vi "Main.vi"() -> ()   [LabVIEW 2020]
uses:
  <vilib>/Utility/error.llb/DialogType.ctl
  <vilib>/DAQmx/read.llb/DAQmx Read (Analog 1D Wfm NChan NSamp).vi
  <extravilib>/ChannelInstances/Tag-bool/Write With Abort.vi
  <extravilib>/ChannelInstances/Tag-bool/Read With Abort.vi
  <extravilib>/ChannelInstances/Tag-bool/Instantiate.vi
  <vilib>/DAQmx/create/channels.llb/DAQmx Create Channel (AI-Acceleration-Accelerometer).vi
  <vilib>/DAQmx/configure/timing.llb/DAQmx Timing (Sample Clock).vi
  <extravilib>/ChannelInstances/Tag-bool/EndpointRead.vi
  <vilib>/DAQmx/miscellaneous.llb/DAQmx Fill In Error Info.vi
  <vilib>/Waveform/DWDTOps.llb/DWDT Digital to Analog.vi
  <vilib>/ULx/Create Channel.llb/ULx Create Channel (AI-Voltage-Basic).vi
  <vilib>/ULx/Timing.llb/ULx Timing (Sample Clock).vi
  <vilib>/ULx/Read.llb/ULx Read (Analog 1D Wfm NChan NSamp).vi
  <vilib>/DAQmx/create/channels.llb/DAQmx Create Channel (CO-Pulse Generation-Frequency).vi
  <vilib>/DAQmx/configure/timing.llb/DAQmx Timing (Implicit).vi
  <extravilib>/ChannelInstances/Tag-bool/Endpoint.vi
  <extravilib>/ChannelInstances/Tag-bool.lvlib
panel:
  in  "Accels":bool
  in  "Tach":bool
  in  "Mic Enable":bool
  in  "Load Enable":bool
  in  "Encoder Enable":bool
  in  "Torque/Power Enable":bool
  in  "Doppler":bool
  out "Feet Traveled":u64
  out "Power":dynamicdata(graph)
  out "Rev Count":u16
  out "Torque":dynamicdata(graph)
  out "Tach Graph":digitalwaveform[](graph)
  out "Accel Graph":waveform(dbl)[](graph)
  out "Microphones":dynamicdata(graph)
  out "Load Cell Graph":waveform(dbl)[](graph)
  in  "stop":bool
  # "Doppler Speed Sensor"
  # "Torque Encoder"
  # "Operation Instructions: Use the toggle buttons to turn on/off the data acquisition for the various sensors. The Power and Torque are aquired together so toggling the Torque button will also toggle Power.\nPress Run from the toolbar (ctrl + r) to start acquisition and press the Stop key to end aquisition. Make sure sensor power supplies are on!!!"
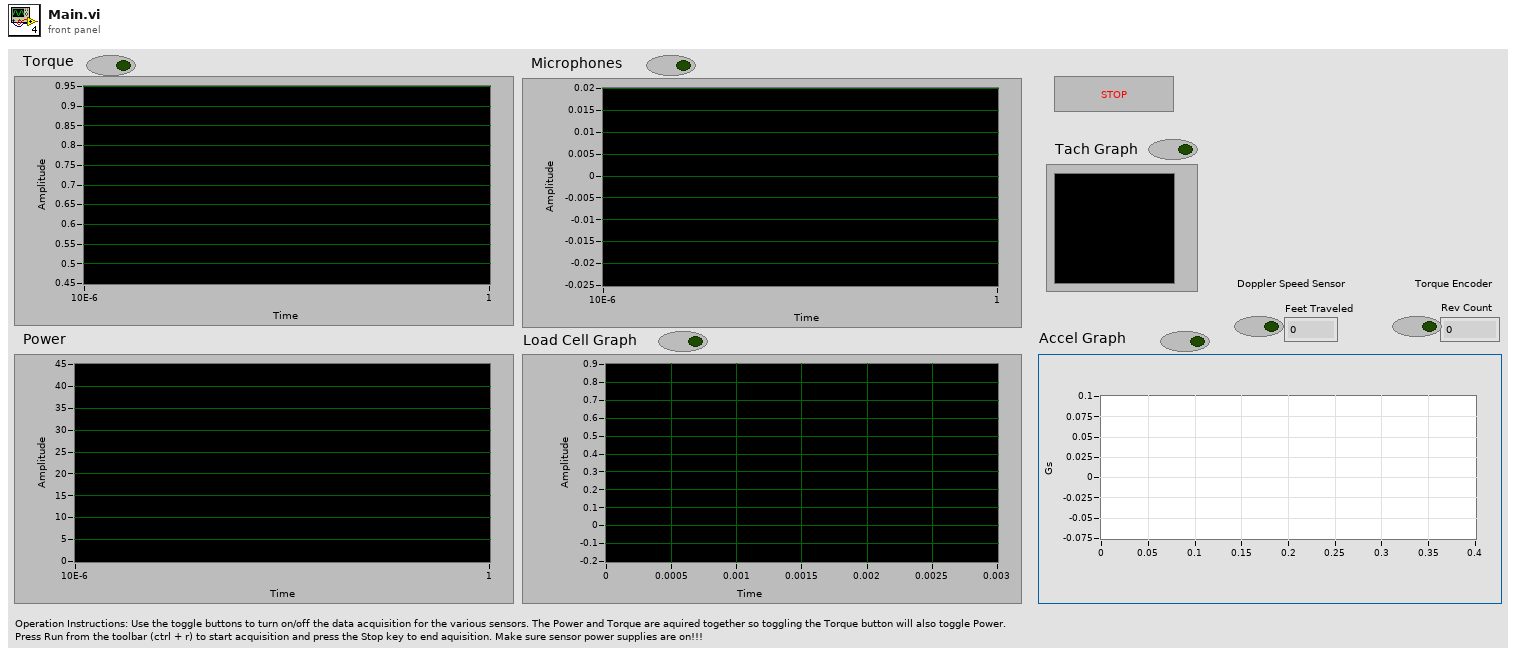
[diagram p1: front panel]
types:
  T1 = typedef "DialogType.ctl" = u16
  T2 = typedef "Tag-bool.lvlib/))Channel.ctl" = refnum<queue>
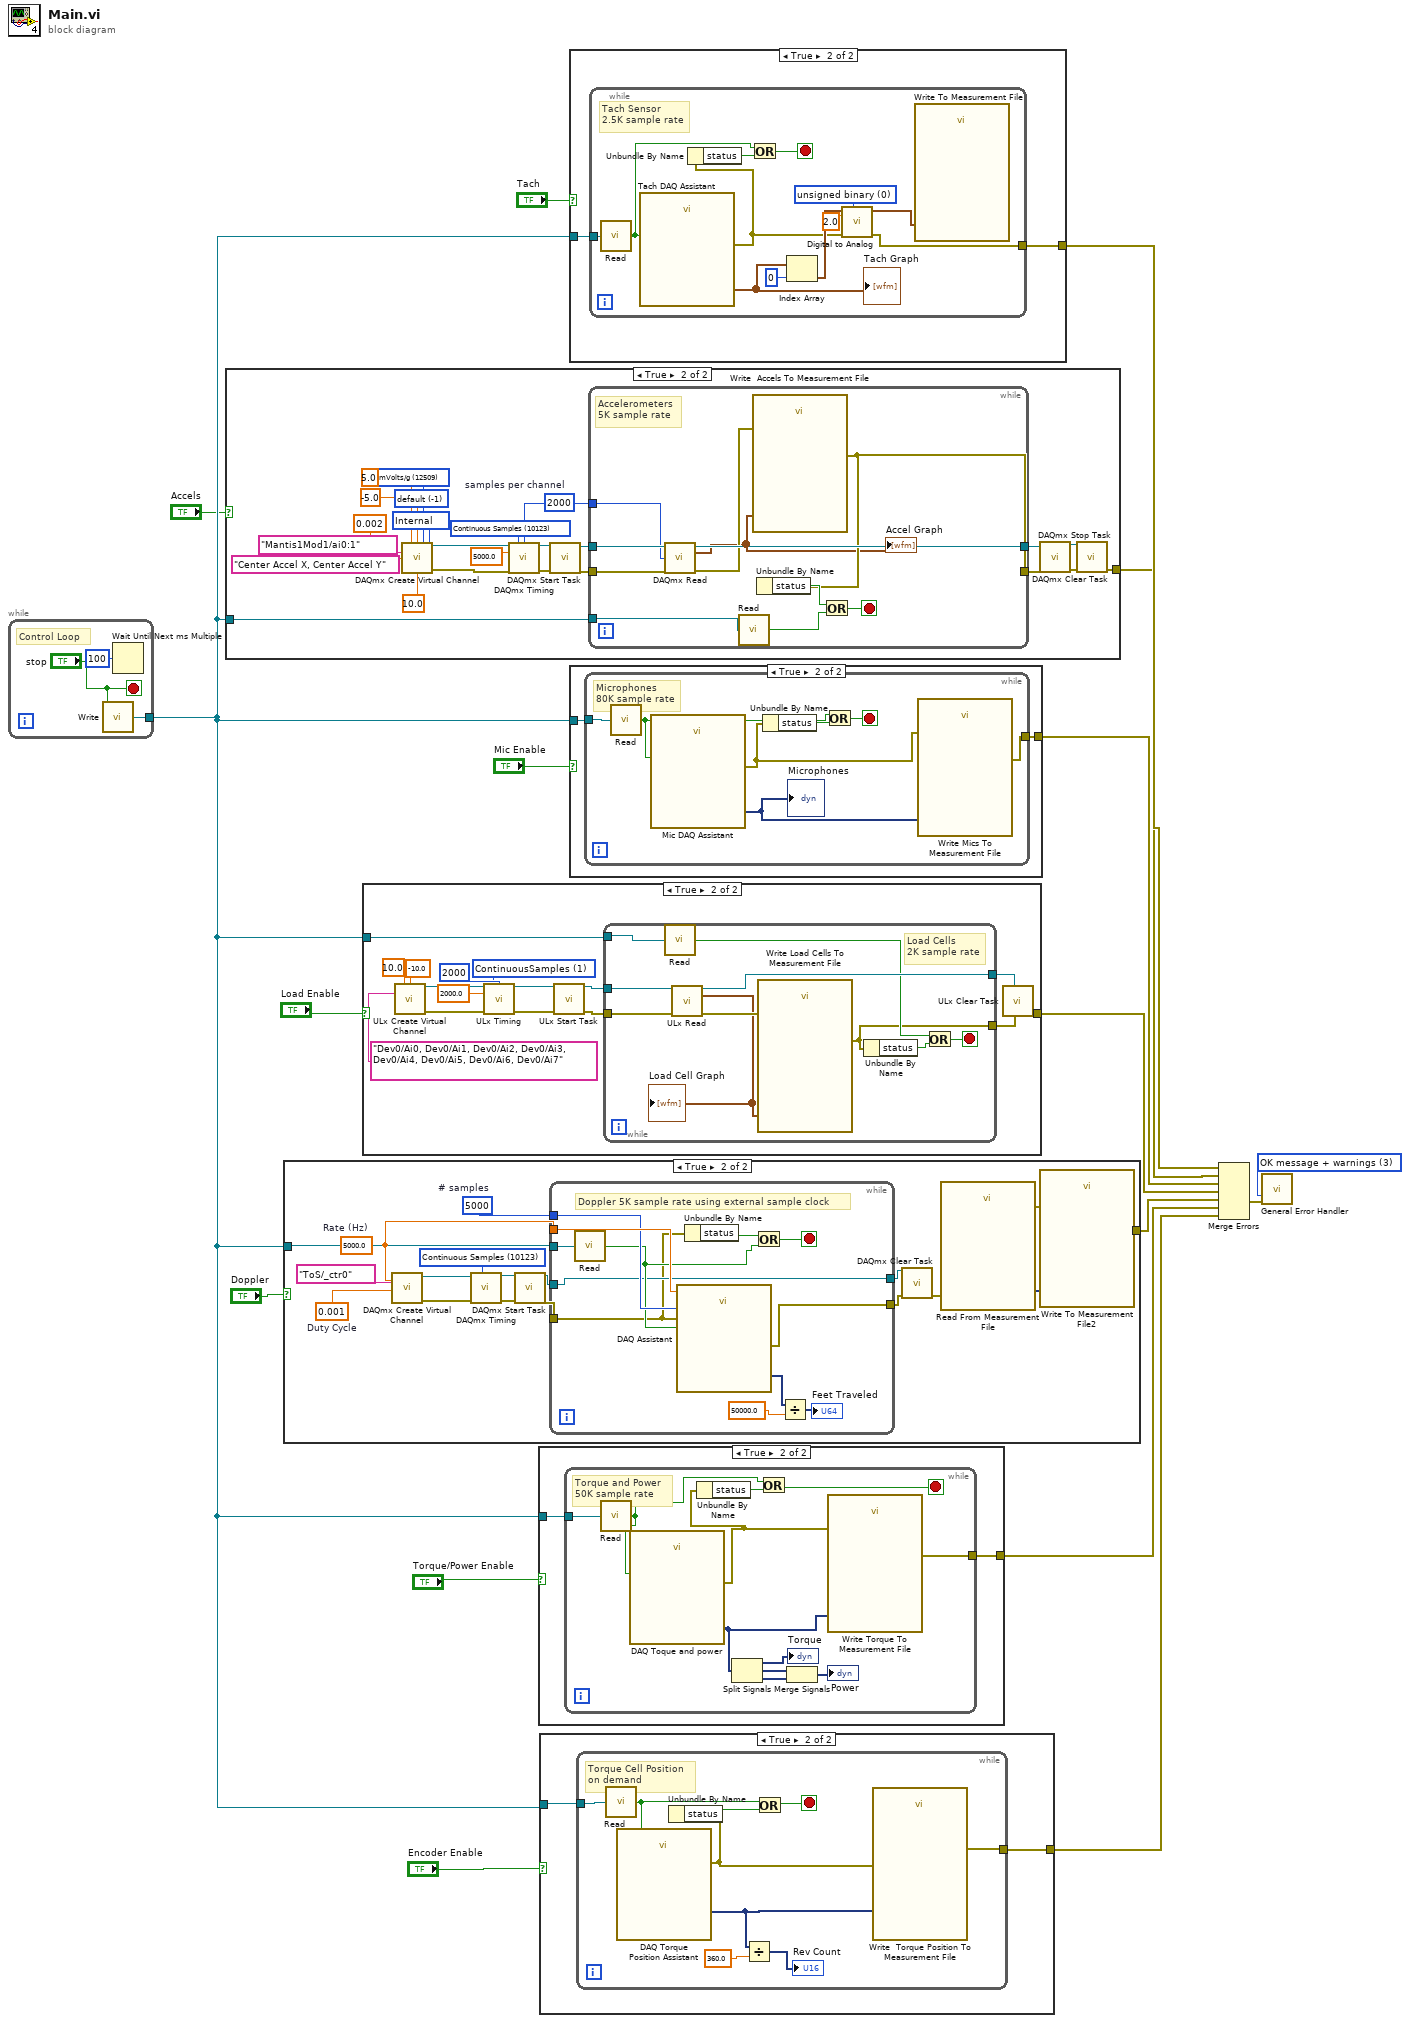
[diagram p0: block diagram]
diagram:
  w17 = T1 3 items=["no dialog", "OK message", "continue or stop message", "OK message + warnings", "continue/stop + warnings"] ("type of dialog (OK msg:1)")
  n1 = while {
    tunnel: [w18] -> w16
    stop <- "stop" stop-if-true
    # "Control Loop"
    n2 = call <extravilib>:"Write.vi"("element"="stop") -> ("channel"=w18:T2)  [unwired: 1 out]
    n3 = Wait Until Next ms Multiple(millisecond multiple=u32 100 ("millisecond timer value")) -> ()  [unwired: 1 out]
  }
  n4 = case shown="True" "Accels" {
    tunnel: w16 -> [_ w22]
    tunnel: [_ w21] -> w7
    frame False {
    }
    frame True {
      w26 = 12509 items=["mVolts/g"=12509, "Volts/g"=12510] ("sensitivity units")
      w29 = 10200 items=["Internal"=10200, "External"=10167, "None"=10230] ("current excitation source")
      w30 = -1 items=["default"=-1, "RSE"=10083, "NRSE"=10078, "Differential"=10106, "Pseudodifferential"=12529] ("input terminal configuration")
      w34 = 2000  # samples per channel
      w42 = 10123 items=["Finite Samples"=10178, "Continuous Samples"=10123, "Hardware Timed Single Point"=12522] ("Sample Mode")
      n5 = call-poly <vilib>:"DAQmx Create Virtual Channel.vi"("maximum value"=5.0, "minimum value"=-5.0, "input terminal configuration"=w30, "physical channels"=tag "Mantis1Mod1/ai0:1", "current excitation source"=w29, "name to assign"="Center Accel X, Center Accel Y", "current excitation value"=0.002, "sensitivity"=10.0, "sensitivity units"=w26) -> ("task out"=w24:refnum<k21>, "error out"=w23:errorcluster)  [unwired: 5 in]
      n6 = call-poly <vilib>:"DAQmx Timing.vi"("task/channels in"=w24, "sample mode"=w42, "samples per channel"=w34, "rate"=5000.0, "error in"=w23) -> ("task out"=w44:refnum<k21>, "error out"=w43:errorcluster)  [unwired: 9 in]
      n7 = call <vilib>:"DAQmx Start Task.vi"("task/channels in"=w44, "error in"=w43) -> ("task out"=w41:refnum<k21>, "error out"=w40:errorcluster)  [unwired: 12 in]
      n8 = while {
        tunnel: w41 -> [w55]
        tunnel: w40 -> [w54]
        tunnel: [w53] -> w39
        tunnel: [w46] -> w38
        tunnel: w34 -> [w50]
        tunnel: w22 -> [w48]
        stop <- w51 stop-if-true
        # "Accelerometers\n5K sample rate"
        n9 = call-poly <vilib>:"DAQmx Read.vi"("task/channels in"=w55, "number of samples per channel"=w50, "error in"=w54) -> ("task out"=w53:refnum<k21>, "data"=w45:waveform(dbl)[], "error out"=w47:errorcluster)  [unwired: 10 in]
        "Accel Graph" <- w45
        n10 = call <extravilib>:"Read.vi"("channel"=w48) -> ("element"=w49:bool)  [unwired: 1 in, 1 out]
        n11 = call "Write  Accels To Measurement File"("Signals"=w45, "error in (no error)"=w47) -> ("error out"=w46:errorcluster)  [unwired: 15 in, 2 out]
        n12 = Unbundle By Name(w46) -> ("status"=w52:bool)
        n13 = Or(x=w52, y=w49) -> (x .or. y?=w51:bool)
      }
      n14 = call <vilib>:"DAQmx Stop Task.vi"("task/channels in"=w39, "error in"=w38) -> ("task out"=w36:refnum<k21>, "error out"=w37:errorcluster)  [unwired: 12 in]
      n15 = call <vilib>:"DAQmx Clear Task.vi"("task in"=w36, "error in"=w37) -> ("error out"=w21:errorcluster)  [unwired: 13 in]
    }
  }
  n16 = case shown="True" "Doppler" {
    tunnel: w16 -> [_ w66]
    tunnel: [_ w59] -> w2
    frame False {
    }
    frame True {
      w68 = 5000  # # samples
      w56 = 5000.0  # Rate (Hz)
      w69 = 0.001  # Duty Cycle
      w71 = 10123 items=["Finite Samples"=10178, "Continuous Samples"=10123] ("sample mode")
      n17 = call-poly <vilib>:"DAQmx Create Virtual Channel.vi"("frequency"=w56, "duty cycle"=w69, "counter"=tag "ToS/_ctr0" ("Sample Clock Src")) -> ("task out"=w72:refnum<k21>, "error out"=w73:errorcluster)  [unwired: 11 in]
      n18 = call-poly <vilib>:"DAQmx Timing.vi"("task/channels in"=w72, "sample mode"=w71, "error in"=w73) -> ("task out"=w58:refnum<k21>, "error out"=w57:errorcluster)  [unwired: 11 in]
      n19 = call <vilib>:"DAQmx Start Task.vi"("task/channels in"=w58, "error in"=w57) -> ("task out"=w63:refnum<k21>, "error out"=w61:errorcluster)  [unwired: 12 in]
      n20 = while {
        tunnel: w56 -> [w85]
        tunnel: w68 -> [w83]
        tunnel: [w81] -> w67
        tunnel: w66 -> [w76]
        tunnel: w63 -> [w75]
        tunnel: [w75] -> w62
        tunnel: w61 -> [w74]
        stop <- w82 stop-if-true
        # "Doppler 5K sample rate using external sample clock"
        n21 = call <extravilib>:"Read.vi"("channel"=w76) -> ("element"=w77:bool)  [unwired: 1 in, 1 out]
        n22 = call "DAQ Assistant"("rate"=w85, "number of samples"=w83, "error in"=w74, "stop (F)"=w77) -> ("data"=w79:dynamicdata, "error out"=w81:errorcluster)  [unwired: 12 in, 2 out]
        n23 = Unbundle By Name(w74) -> ("status"=w84:bool)
        n24 = Or(x=w84, y=w77) -> (x .or. y?=w82:bool)
        n25 = Divide(x=w79, y=50000.0) -> (x/y=→"Feet Traveled":dynamicdata)
      }
      n26 = call <vilib>:"DAQmx Clear Task.vi"("task in"=w62, "error in"=w67) -> ("error out"=w60:errorcluster)  [unwired: 13 in]
      n27 = call "Read From Measurement File"("error in (no error)"=w60) -> ("error out"=w64:errorcluster, "Signals"=w65:dynamicdata)  [unwired: 5 in, 4 out]
      n28 = call "Write To Measurement File2"("Signals"=w65, "error in (no error)"=w64) -> ("error out"=w59:errorcluster)  [unwired: 15 in, 2 out]
    }
  }
  n29 = case shown="True" "Load Enable" {
    tunnel: w16 -> [_ w87]
    tunnel: [_ w86] -> w14
    frame False {
    }
    frame True {
      w94 = 1 items=["FiniteSamples", "ContinuousSamples"] ("sample mode")
      n30 = call-poly <vilib>:"ULx Create Virtual Channel.vi"("maximum value"=10.0, "minimum value"=-10.0, "physical channels"="Dev0/Ai0, Dev0/Ai1, Dev0/Ai2, Dev0/Ai3, Dev0/Ai4, Dev0/Ai5, Dev0/Ai6, Dev0/Ai7") -> ("task out"=w99:refnum<k24>, "error out"=w101:errorcluster)  [unwired: 11 in]
      n31 = call-poly <vilib>:"ULx Timing.vi"("task in"=w99, "sample mode"=w94, "samples per channel"=2000, "rate"=2000.0, "error in"=w101) -> ("task out"=w90:refnum<k24>, "error out"=w97:errorcluster)  [unwired: 9 in]
      n32 = call <vilib>:"ULx Start Task.vi"("task in"=w90, "error in"=w97) -> ("task out"=w98:refnum<k24>, "error out"=w100:errorcluster)  [unwired: 12 in]
      n33 = while {
        tunnel: w100 -> [w108]
        tunnel: w98 -> [w111]
        tunnel: [w110] -> w89
        tunnel: w87 -> [w107]
        tunnel: [w103] -> w88
        stop <- w109 stop-if-true
        # "Load Cells\n2K sample rate"
        n34 = call <extravilib>:"Read.vi"("channel"=w107) -> ("element"=w105:bool)  [unwired: 1 in, 1 out]
        n35 = call-poly <vilib>:"ULx Read.vi"("task in"=w111, "error in"=w108) -> ("task out"=w110:refnum<k24>, "data"=w102:waveform(dbl)[], "error out"=w104:errorcluster)  [unwired: 11 in]
        "Load Cell Graph" <- w102
        n36 = call "Write Load Cells To Measurement File"("Signals"=w102, "error in (no error)"=w104) -> ("error out"=w103:errorcluster)  [unwired: 15 in, 2 out]
        n37 = Unbundle By Name(w103) -> ("status"=w106:bool)
        n38 = Or(x=w105, y=w106) -> (x .or. y?=w109:bool)
      }
      n39 = call <vilib>:"ULx Clear Task.vi"("task in"=w89, "error in"=w88) -> ("error out"=w86:errorcluster)  [unwired: 13 in]
    }
  }
  n40 = case shown="True" "Torque/Power Enable" {
    tunnel: w16 -> [_ w113]
    tunnel: [_ w112] -> w1
    frame False {
    }
    frame True {
      n41 = while {
        tunnel: w113 -> [w124]
        tunnel: [w119] -> w112
        stop <- w122 stop-if-true
        # "Torque and Power\n50K sample rate"
        n42 = call <extravilib>:"Read.vi"("channel"=w124) -> ("element"=w121:bool)  [unwired: 1 in, 1 out]
        n43 = call "DAQ Toque and power"("stop (F)"=w121) -> ("data"=w118:dynamicdata, "error out"=w120:errorcluster)  [unwired: 15 in, 2 out]
        n44 = Unbundle By Name(w120) -> ("status"=w123:bool)
        n45 = Split Signals(w118) -> (→"Torque":dynamicdata, w116:dynamicdata, w115:dynamicdata)  [unwired: 3 in]
        n46 = Or(x=w121, y=w123) -> (x .or. y?=w122:bool)
        n47 = Merge Signals(w116, w115) -> (→"Power":dynamicdata)
        n48 = call "Write Torque To Measurement File"("Signals"=w118, "error in (no error)"=w120) -> ("error out"=w119:errorcluster)  [unwired: 15 in, 2 out]
      }
    }
  }
  n49 = case shown="True" "Encoder Enable" {
    tunnel: w16 -> [_ w126]
    tunnel: [_ w125] -> w13
    frame False {
    }
    frame True {
      n50 = while {
        tunnel: w126 -> [w131]
        tunnel: [w130] -> w125
        stop <- w135 stop-if-true
        # "Torque Cell Position\non demand"
        n51 = call <extravilib>:"Read.vi"("channel"=w131) -> ("element"=w132:bool)  [unwired: 1 in, 1 out]
        n52 = call "DAQ Torque Position Assistant"("stop (F)"=w132) -> ("data"=w129:dynamicdata, "error out"=w133:errorcluster)  [unwired: 15 in, 2 out]
        n53 = Unbundle By Name(w133) -> ("status"=w134:bool)
        n54 = Divide(x=w129, y=360.0) -> (x/y=→"Rev Count":dynamicdata)
        n55 = Or(x=w132, y=w134) -> (x .or. y?=w135:bool)
        n56 = call "Write  Torque Position To Measurement File"("Signals"=w129, "error in (no error)"=w133) -> ("error out"=w130:errorcluster)  [unwired: 15 in, 2 out]
      }
    }
  }
  n57 = case shown="True" "Tach" {
    tunnel: w16 -> [_ w137]
    tunnel: [_ w136] -> w8
    frame False {
    }
    frame True {
      n58 = while {
        tunnel: w137 -> [w149]
        tunnel: [w140] -> w136
        stop <- w148 stop-if-true
        w142 = u16 0 items=["unsigned binary", "offset binary", "2's complement"] ("data format (offset binary)")
        # "Tach Sensor\n2.5K sample rate"
        n59 = call <extravilib>:"Read.vi"("channel"=w149) -> ("element"=w146:bool)  [unwired: 1 in, 1 out]
        n60 = call "Tach DAQ Assistant"("stop (F)"=w146) -> ("data"=w145:digitalwaveform[], "error out"=w141:errorcluster)  [unwired: 15 in, 2 out]
        "Tach Graph" <- w145
        n61 = Unbundle By Name(w141) -> ("status"=w147:bool)
        n62 = Or(x=w146, y=w147) -> (x .or. y?=w148:bool)
        n63 = Index Array(array=w145, index=0) -> (element=w143:digitalwaveform)
        n64 = call-poly <vilib>:"Digital to Analog.vi"("data format (offset binary)"=w142, "error in (no error)"=w141, "full-scale range (pk-pk)"=2.0, "digital waveform"=w143) -> ("error out"=w140:errorcluster, "analog waveform"=w139:waveform(dbl))  [unwired: 4 in, 2 out]
        n65 = call "Write To Measurement File"("Signals"=w139) -> ()  [unwired: 16 in, 3 out]
      }
    }
  }
  n66 = case shown="True" "Mic Enable" {
    tunnel: w16 -> [_ w151]
    tunnel: [_ w150] -> w6
    frame False {
    }
    frame True {
      n67 = while {
        tunnel: w151 -> [w158]
        tunnel: [w154] -> w150
        stop <- w157 stop-if-true
        # "Microphones\n80K sample rate"
        n68 = call <extravilib>:"Read.vi"("channel"=w158) -> ("element"=w156:bool)  [unwired: 1 in, 1 out]
        n69 = call "Mic DAQ Assistant"("stop (F)"=w156) -> ("data"=w153:dynamicdata, "error out"=w152:errorcluster)  [unwired: 15 in, 2 out]
        "Microphones" <- w153
        n70 = Unbundle By Name(w152) -> ("status"=w155:bool)
        n71 = Or(x=w156, y=w155) -> (x .or. y?=w157:bool)
        n72 = call "Write Mics To Measurement File"("Signals"=w153, "error in (no error)"=w152) -> ("error out"=w154:errorcluster)  [unwired: 15 in, 2 out]
      }
    }
  }
  n73 = Merge Errors(w8, w7, w6, w14, w2, w1, w13) -> (w15:errorcluster)
  n74 = call <vilib>:"General Error Handler.vi"("type of dialog (OK msg:1)"=w17, "error in (no error)"=w15) -> ()  [unwired: 9 in, 5 out]
